vi "Pack Message.vi"(8 "error in (no error)":errorcluster, 11 "Message Double in":refnum<class "Message 2D String Array.lvclass">) -> (0 "error out":errorcluster, 1 "Packed Message":string, 2 "Message Name":string, 3 "Message Double out":refnum<class "Message 2D String Array.lvclass">)   [LabVIEW 2016, in "WebSocket Networking.lvlib" / "Message 2D String Array.lvclass"]
uses:
  <userlib>/Common Components/WebSocket Networking/Message 2D String Array/Message 2D String Array.lvclass
  C:/Program Files (x86)/National Instruments/LabVIEW 2016/user.lib/Composed Systems/Stream/Mediator/Classes/Message Interface/Message Interface.lvclass
  <userlib>/Common Components/WebSocket Networking/Message 2D String Array/Message 2D String Array.lvclass/Message 2D String Array.ctl
  <userlib>/Composed Systems/Stream/Mediator/Classes/Message Interface/Message Interface.lvclass
  <vilib>/addons/_JKI.lib/Serialization/JSON/JKI JSON Serialization.lvlib
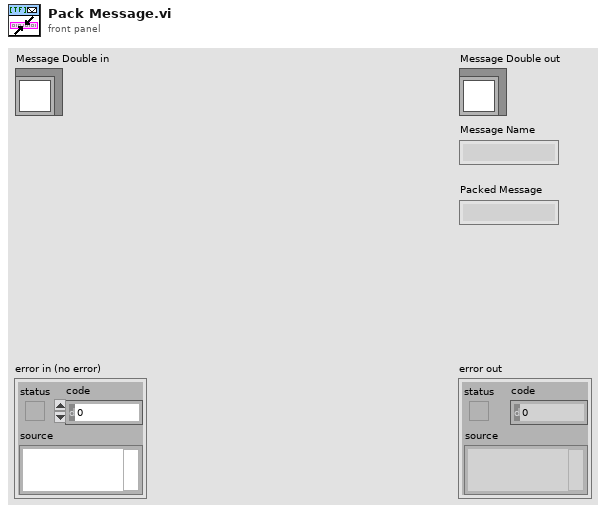
[diagram p1: front panel]
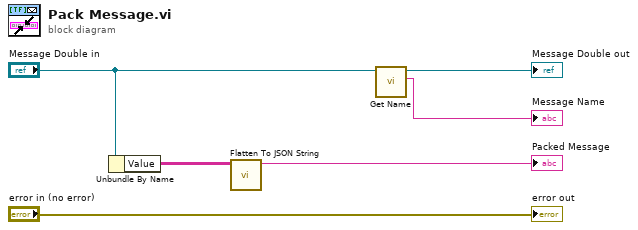
[diagram p0: block diagram]
diagram:
  n1 = Unbundle By Name("Message Double in") -> ("Value"=w2:string[][])
  n2 = call <vilib>:"Flatten To JSON String.vi"("Variant"=w2) -> ("JSON String"=→"Packed Message":string)  [unwired: 9 in, 1 out]
  n3 = call <userlib>:"Get Name.vi"("Message Interface in"="Message Double in") -> ("Name"=→"Message Name":string, "Message Interface out"=→"Message Double out":refnum<class "Message 2D String Array.lvclass">)  [unwired: 8 in, 1 out]
  "error out" <- "error in (no error)"
